vi "Optionen Cluster Initialisieren.vi"(6 "Sprachliste":string[][](array[string]), 7 "Optionen":T1, 8 "error in (no error)":errorcluster caption="Fehler (Eingang, kein Fehler)", 9 "PWL9":bool[](array[boolean]), 10 "sichtbar":bool[](array[boolean]), 11 "Cluster (Eingang)":refnum<vi>) -> (0 "error out":errorcluster caption="Fehler (Ausgang)", 2 "Numerisch 2":i32, 3 "Numerisch":i32)   [LabVIEW 2020, in "System Einstellungen V2.lvlib"]
uses:
  System Einstellungen V2.lvlib
  Optionen.ctl
  Passwortverwaltung/FGV Passwort Aktion.ctl
  Passwortverwaltung/Passwort.lvlib
  Sprachverwaltung/Sprachverwaltung.lvlib
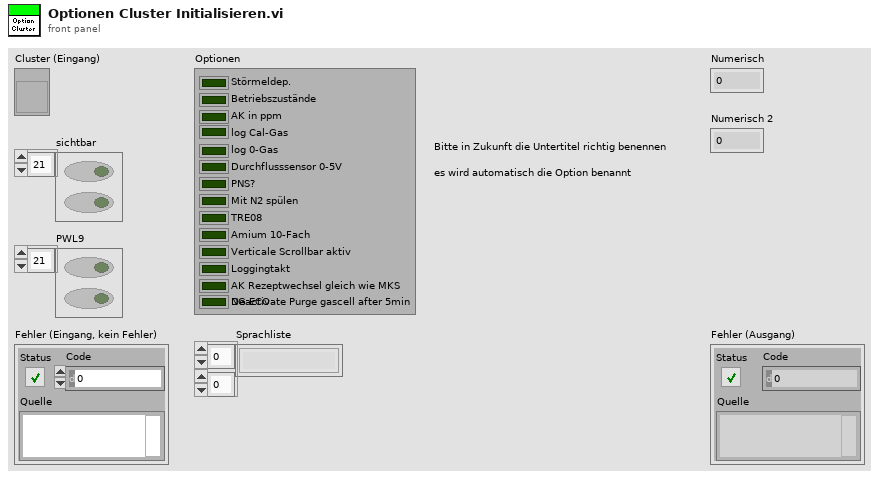
[diagram p1: front panel]
types:
  T1 = typedef "System Einstellungen V2.lvlib/Optionen.ctl" = cluster{"Störmeldep.":bool, "Betriebszustände":bool, "AK in ppm":bool, "log Cal-Gas":bool, "log 0-Gas":bool, "Durchflusssensor 0-5V":bool, "PNS?":bool, "Mit N2 spülen":bool, "TRE08":bool, "Amium 10-Fach":bool, "Verticale Scrollbar aktiv":bool, "Loggingtakt":bool, "AK Rezeptwechsel gleich wie MKS":bool, "NG ECO":bool}
  T2 = typedef "Passwort.lvlib/FGV Passwort Aktion.ctl" = enum16{"prüfen", "setzen", "Initialisieren", "PW speichern", "lesen", "PW Änderung"}
  T3 = enum8{"Enabled", "Disabled", "Disabled and Grayed Out"}
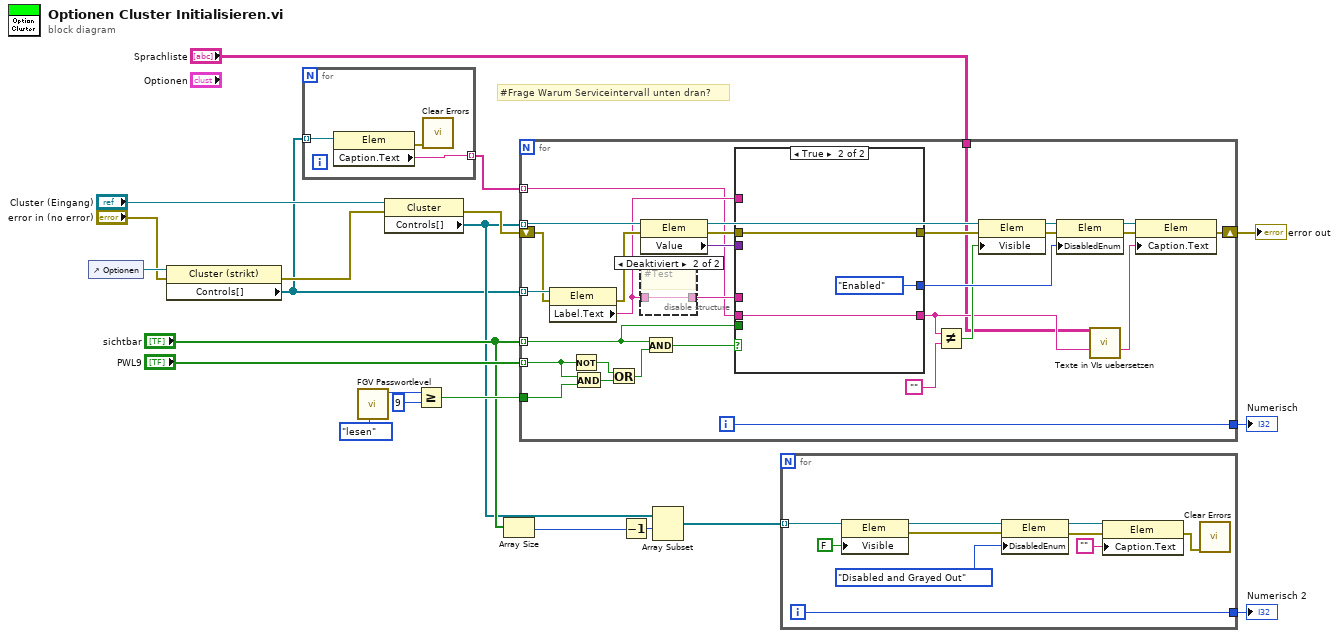
[diagram p0: block diagram]
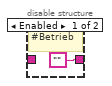
[diagram p2: hidden frame]
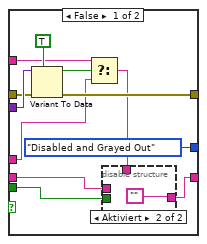
[diagram p3: hidden frame]
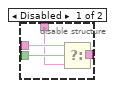
[diagram p4: hidden frame]
diagram:
  # "#Frage Warum Serviceintervall unten dran?"
  n1 = control-ref of="Optionen"() -> (w6:refnum<vi>)
  n2 = property class="Cluster (strikt)"(reference=w6, error in="error in (no error)") -> (error out=w4:errorcluster, "Controls[]"=w3:refnum<vi>[])  [unwired: 1 out]
  n3 = for {
    tunnel: w3 -> [w24] mode=indexing
    tunnel: [w23] -> w2 mode=indexing
    n4 = property class="Elem"(reference=w24) -> (error out=w22:errorcluster, "Caption.Text"=w23:string)  [unwired: 1 in, 1 out]
    n5 = call <vilib>:"Clear Errors.vi"("error in (no error)"=w22) -> ()  [unwired: 5 in, 2 out]
  }
  n6 = call "FGV Passwortlevel.vi"("FGV Passwort Aktion"=FGV_Passwort_Aktion."lesen") -> ("aktueller Level"=w17:i16)  [unwired: 8 in, 2 out]
  n7 = property class="Cluster"(reference="Cluster (Eingang)", error in=w4) -> (error out=w20:errorcluster, "Controls[]"=w12:refnum<vi>[])  [unwired: 1 out]
  n8 = Greater Or Equal?(x=w17, y=i16 9) -> (x >= y?=w15:bool)
  n9 = Array Size(array="sichtbar") -> (size(s)=w11:i32)
  n10 = for {
    tunnel: "sichtbar" -> [w43] mode=indexing
    tunnel: w12 -> [w41] mode=indexing
    shift-right: [w53] -> w19
    shift-left: w20 -> [w38]
    tunnel: w15 -> [w52]
    tunnel: "PWL9" -> [w49] mode=indexing
    tunnel: [w42] -> w9
    tunnel: w3 -> [w39] mode=indexing
    tunnel: w2 -> [w28] mode=indexing
    tunnel: "Sprachliste" -> [w25]
    i -> [w42]
    n11 = property class="Elem"(reference=w39, error in=w38) -> (error out=w37:errorcluster, "Label.Text"=w30:string)  [unwired: 1 out]
    n12 = Not(x=w49) -> (.not. x?=w48:bool)
    n13 = And(x=w49, y=w52) -> (x .and. y?=w51:bool)
    n14 = Or(x=w48, y=w51) -> (x .or. y?=w50:bool)
    n15 = property class="Elem"(reference=w41, error in=w37) -> (reference out=w40:refnum<vi>, error out=w32:errorcluster, "Value"=w36:variant)
    n16 = disable-structure shown="Deaktiviert" {
      disable-tunnel: w30 -> [_ w56]
      disable-tunnel: ["" w56] -> w35
      frame Enabled {
        # "#Betrieb"
      }
      frame Disabled {
        # "#Test"
      }
    }
    n17 = And(x=w43, y=w50) -> (x .and. y?=w46:bool)
    n18 = case shown="True" w46 {
      tunnel: [T3."Disabled and Grayed Out" ("Deaktiviert") T3."Enabled" ("Deaktiviert")] -> w47
      tunnel: w28 -> [w66 w75]
      tunnel: [w65 w75] -> w27
      tunnel: w43 -> [w67 _]
      tunnel: w35 -> [w59 _]
      tunnel: w36 -> [w63 _]
      tunnel: w32 -> [w62 w74]
      tunnel: [w61 w74] -> w31
      tunnel: w30 -> [w57 _]
      frame False {
        n19 = Variant To Data(error in=w62, type=TRUE, Variant=w63) -> (data=w60:bool, error out=w61:errorcluster)
        n20 = Select(t=w57, s=w60, f=w59) -> (s? t:f=w58:string)
        n21 = disable-structure shown="Aktiviert" {
          disable-tunnel: w67 -> [w72 _]
          disable-tunnel: w66 -> [w71 _]
          disable-tunnel: [w70 ""] -> w65
          disable-tunnel: w58 -> [w69 _]
          frame Disabled {
            n22 = Select(t=w71, s=w72, f=w69) -> (s? t:f=w70:string)
          }
          frame Enabled {
          }
        }
      }
      frame True {
      }
    }
    n23 = Not Equal?(x=w27, y="") -> (x != y?=w33:bool)
    n24 = property class="Elem"(reference=w40, error in=w31, "Visible"=w33) -> (reference out=w44:refnum<vi>, error out=w45:errorcluster)
    n25 = property class="Elem"(reference=w44, error in=w45, "DisabledEnum"=w47) -> (reference out=w54:refnum<vi>, error out=w29:errorcluster)
    n26 = call "Texte in VIs uebersetzen.vi"("Sprachliste"=w25, "String zum Übersetzen"=w27) -> ("String zum Übersetzen"=w26:string)  [unwired: 9 in, 4 out]
    n27 = property class="Elem"(reference=w54, error in=w29, "Caption.Text"=w26) -> (error out=w53:errorcluster)  [unwired: 1 out]
  }
  "error out" <- w19
  "Numerisch" <- w9
  n28 = Decrement(x=w11) -> (x-1=w7:i32)
  n29 = Array Subset(array=w12, index=w7) -> (w10:refnum<vi>[])  [unwired: 1 in]
  n30 = for {
    tunnel: w10 -> [w81] mode=indexing
    tunnel: [w77] -> w8
    i -> [w77]
    n31 = property class="Elem"(reference=w81, "Visible"=FALSE ("Sichtbar")) -> (reference out=w80:refnum<vi>, error out=w79:errorcluster)  [unwired: 1 in]
    n32 = property class="Elem"(reference=w80, error in=w79, "DisabledEnum"=T3."Disabled and Grayed Out" ("Deaktiviert")) -> (reference out=w86:refnum<vi>, error out=w85:errorcluster)
    n33 = property class="Elem"(reference=w86, error in=w85, "Caption.Text"="") -> (error out=w84:errorcluster)  [unwired: 1 out]
    n34 = call <vilib>:"Clear Errors.vi"("error in (no error)"=w84) -> ()  [unwired: 5 in, 2 out]
  }
  "Numerisch 2" <- w8
